vi "GetCustomDeviceInitializationVI.vi"(8 "error in (no error)":errorcluster, 11 "custom device reference in":refnum<k24>) -> (0 "error out":errorcluster, 2 "initialization VI":T1, 3 "custom device reference out":refnum<k24>)   [LabVIEW 2017, in "VeriStandTestUtilities.lvlib"]
uses:
  VeriStandTestUtilities.lvlib
  NationalInstruments.VeriStand.XMLReader
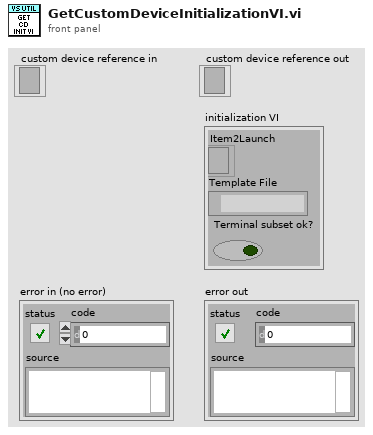
[diagram p1: front panel]
types:
  T1 = cluster{"Item2Launch":refnum<k24>, "Template File":path, "Terminal subset ok?":bool}
  T2 = cluster{"Item2Launch":refnum<k24>, "Template File":path, bool}
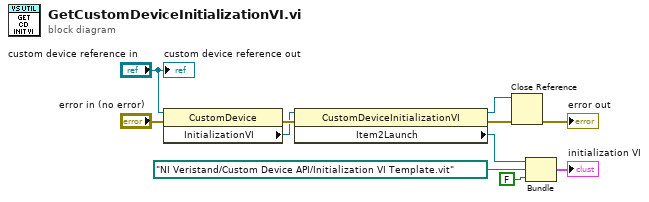
[diagram p0: block diagram]
diagram:
  n1 = property class="CustomDevice"(reference="custom device reference in", error in="error in (no error)") -> (error out=w10:errorcluster, "InitializationVI"=w9:refnum<k24>)  [unwired: 1 out]
  n2 = property class="CustomDeviceInitializationVI"(reference=w9, error in=w10) -> (reference out=w3:refnum<k24>, error out=w8:errorcluster, "Item2Launch"=w5:refnum<k24>)
  n3 = Close Reference(reference=w3, error in (no error)=w8) -> (error out=→"error out":errorcluster)
  n4 = Bundle("Item2Launch"=w5, "Template File"=path "NI Veristand/Custom Device API/Initialization VI Template.vit", FALSE) -> (→"initialization VI":T2)  [unwired: 1 in]
  "custom device reference out" <- "custom device reference in"
